vi "DMM Configuration - Update DMM Measurements ComboBox.vi"(8 "error in (no error)":errorcluster, 9 "DMM Temp - Value In":T1={"DMM Temp - Transducer Type"=1, "DMM Temp - Thermocouple Type"=6, "DMM Temp - Fixed Reference Junction"=25.0, "DMM Temp - RTD Type"=enum."Pt3851", "DMM Temp - RTD Resistance"=100.0, "DMM Temp - Thermistor Type"=enum."44006", "DMM Temp - RTD A"=0.0039083, "DMM Temp - RTD B"=-5.775e-07, "DMM Temp - RTD C"=-4.183e-12, "DMM Temp - Thermistor A"=0.0010295, "DMM Temp - Thermistor B"=0.0002391, "DMM Temp - Thermistor C"=1.568e-07} {"DMM Temp - Thermistor C" format="%#_13g"; "DMM Temp - Thermistor B" format="%#_13g"; "DMM Temp - Thermistor A" format="%#_13g"; "DMM Temp - RTD Resistance" format="%.2f"; "DMM Temp - Fixed Reference Junction" format="%.2f"; "DMM Temp - Thermocouple Type" items=["B"=1, "E"=4, "J"=6, "K"=7, "N"=8, "R"=9, "S"=10, "T"=11]; "DMM Temp - Transducer Type" items=["Thermocouple"=1, "Thermistor"=2, "2-Wire RTD"=3, "4-Wire RTD"=4]}, 10 "Measurement In":T7 caption="Function", 11 "Measurement Controls Refs In":T6) -> (0 "error out":errorcluster, 1 "DMM Temp - Value Out":T1={"DMM Temp - Transducer Type"=1, "DMM Temp - Thermocouple Type"=6, "DMM Temp - Fixed Reference Junction"=25.0, "DMM Temp - RTD Type"=enum."Pt3851", "DMM Temp - RTD Resistance"=100.0, "DMM Temp - Thermistor Type"=enum."44006", "DMM Temp - RTD A"=0.0039083, "DMM Temp - RTD B"=-5.775e-07, "DMM Temp - RTD C"=-4.183e-12, "DMM Temp - Thermistor A"=0.0010295, "DMM Temp - Thermistor B"=0.0002391, "DMM Temp - Thermistor C"=1.568e-07} {"DMM Temp - Thermistor C" format="%#_13g"; "DMM Temp - Thermistor B" format="%#_13g"; "DMM Temp - Thermistor A" format="%#_13g"; "DMM Temp - RTD Resistance" format="%.2f"; "DMM Temp - Fixed Reference Junction" format="%.2f"; "DMM Temp - Thermocouple Type" items=["B"=1, "E"=4, "J"=6, "K"=7, "N"=8, "R"=9, "S"=10, "T"=11]; "DMM Temp - Transducer Type" items=["Thermocouple"=1, "Thermistor"=2, "2-Wire RTD"=3, "4-Wire RTD"=4]}, 2 "Temp Meas?":bool, 3 "Measurement Controls Refs Out":T6)   [LabVIEW 2016, in "DMM-SWITCH-ScanList System Explorer.lvlib"]
uses:
  DMM-SWITCH-ScanList System Explorer.lvlib
  <instrlib>/niDMM/nidmm.llb/niDMM Function.ctl
  Configuration Controls/DMM Temp.ctl
  <instrlib>/niDMM/nidmm.llb/niDMM Transducer Type.ctl
  <instrlib>/niDMM/nidmm.llb/niDMM Thermocouple Type.ctl
  <instrlib>/niDMM/nidmm.llb/niDMM RTD Type.ctl
  <instrlib>/niDMM/nidmm.llb/niDMM Thermistor Type.ctl
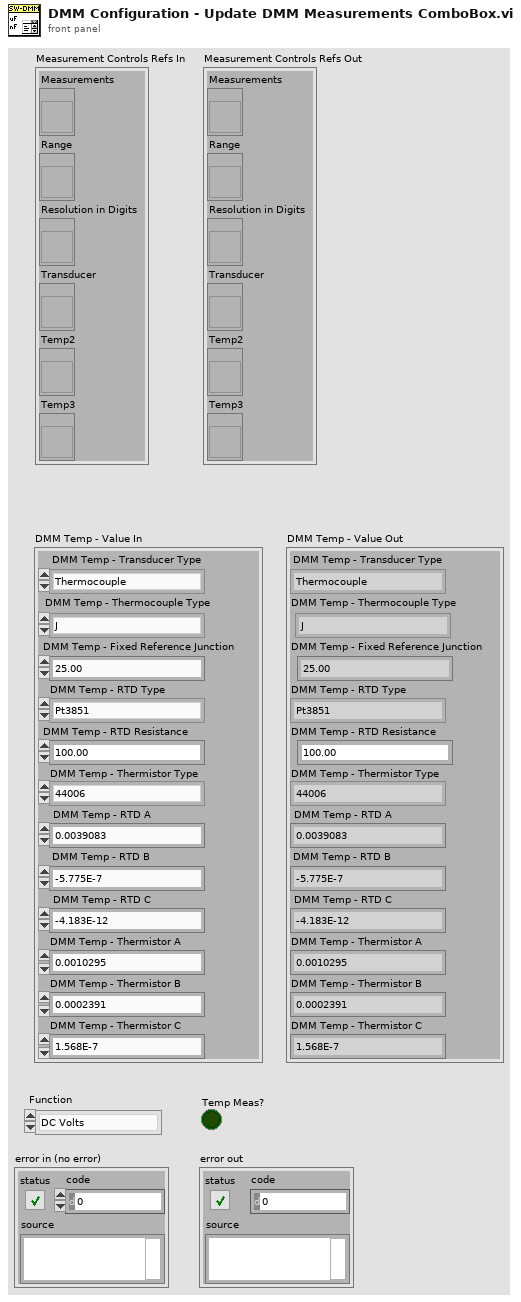
[diagram p1: front panel]
types:
  T1 = typedef "DMM-SWITCH-ScanList System Explorer.lvlib/DMM Temp.ctl" = cluster{"DMM Temp - Transducer Type":T2, "DMM Temp - Thermocouple Type":T3, "DMM Temp - Fixed Reference Junction":dbl, "DMM Temp - RTD Type":T4, "DMM Temp - RTD Resistance":dbl, "DMM Temp - Thermistor Type":T5, "DMM Temp - RTD A":dbl, "DMM Temp - RTD B":dbl, "DMM Temp - RTD C":dbl, "DMM Temp - Thermistor A":dbl, "DMM Temp - Thermistor B":dbl, "DMM Temp - Thermistor C":dbl}
  T2 = typedef "niDMM Transducer Type.ctl" = i32
  T3 = typedef "niDMM Thermocouple Type.ctl" = i32
  T4 = typedef "niDMM RTD Type.ctl" = enum16{"Custom", "Pt3750", "Pt3851", "Pt3911", "Pt3916", "Pt3920", "Pt3928"}
  T5 = typedef "niDMM Thermistor Type.ctl" = enum16{"Custom", "44004", "44006", "44007"}
  T6 = cluster{"Measurements":refnum<vi>, "Range":refnum<vi>, "Resolution in Digits":refnum<vi>, "Transducer":refnum<vi>, "Temp2":refnum<vi>, "Temp3":refnum<vi>}
  T7 = typedef "niDMM Function.ctl" = enum16{"DC Volts", "AC Volts", "DC Current", "AC Current", "2-wire Resistance", "4-wire Resistance", "Diode", "Frequency", "Period", "AC Volts DC Coupled", "Capacitance", "Inductance", "Temperature"}
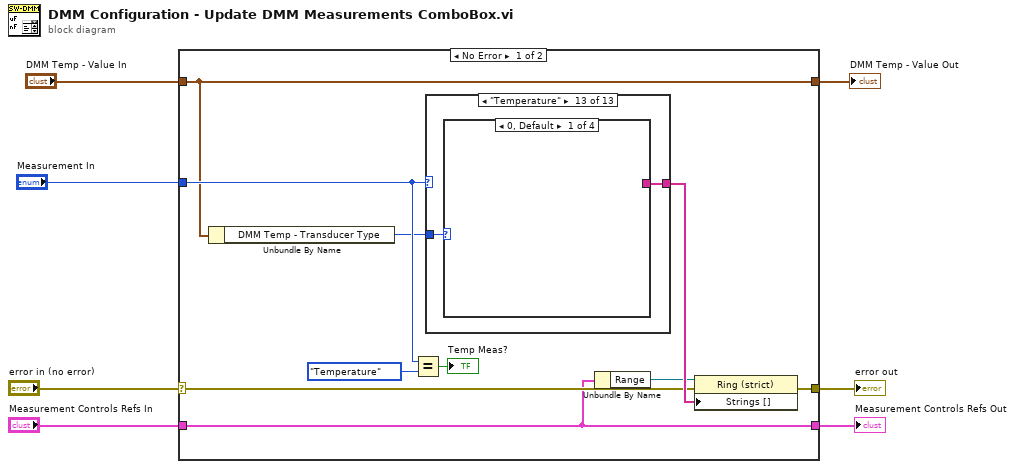
[diagram p0: block diagram]
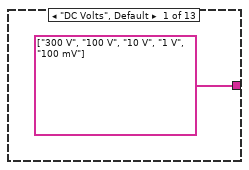
[diagram p2: hidden frame]
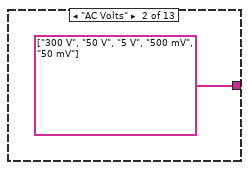
[diagram p3: hidden frame]
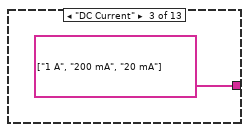
[diagram p4: hidden frame]
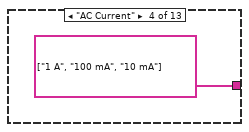
[diagram p5: hidden frame]
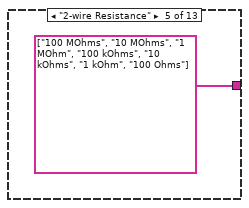
[diagram p6: hidden frame]
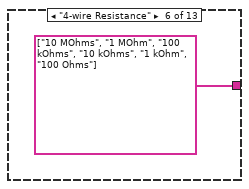
[diagram p7: hidden frame]
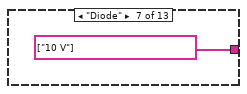
[diagram p8: hidden frame]
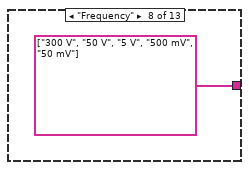
[diagram p9: hidden frame]
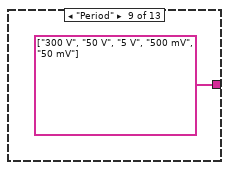
[diagram p10: hidden frame]
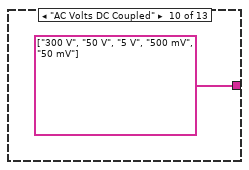
[diagram p11: hidden frame]
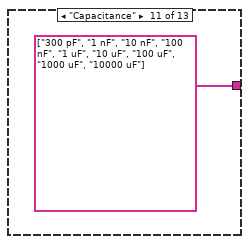
[diagram p12: hidden frame]
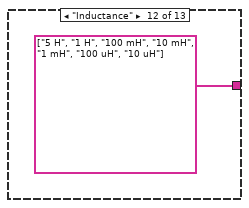
[diagram p13: hidden frame]
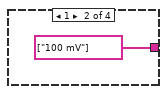
[diagram p14: hidden frame]
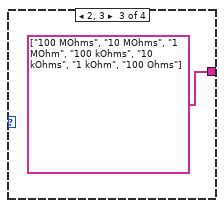
[diagram p15: hidden frame]
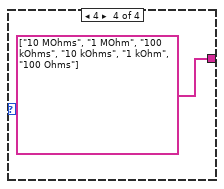
[diagram p16: hidden frame]
diagram:
  n1 = case shown="No Error" "error in (no error)" {
    selector: "error in (no error)" -> [w16 w37]
    tunnel: [w12 w37] -> w7
    tunnel: "Measurement Controls Refs In" -> [w11 w36]
    tunnel: [w11 w36] -> w4
    tunnel: "DMM Temp - Value In" -> [w8 w35]
    tunnel: "Measurement In" -> [w10 _]
    tunnel: [w8 w35] -> w1
    frame No Error {
      n2 = Unbundle By Name(w8) -> ("DMM Temp - Transducer Type"=w9:T2)
      n3 = Equal?(x=w10, y=niDMM_Function."Temperature") -> (x = y?=→"Temp Meas?":bool)
      n4 = case shown="\"Temperature\"" w10 {
        tunnel: [string[] ["300 V", "100 V", "10 V", "1 V", "100 mV"] ("Strings []") string[] ["300 V", "50 V", "5 V", "500 mV", "50 mV"] ("Strings []") string[] ["1 A", "200 mA", "20 mA"] ("Strings []") string[] ["1 A", "100 mA", "10 mA"] ("Strings []") string[] ["100 MOhms", "10 MOhms", "1 MOhm", "100 kOhms", "10 kOhms", "1 kOhm", "100 Ohms"] ("Strings []") string[] ["10 MOhms", "1 MOhm", "100 kOhms", "10 kOhms", "1 kOhm", "100 Ohms"] ("Strings []") string[] ["10 V"] ("Strings []") string[] ["300 V", "50 V", "5 V", "500 mV", "50 mV"] ("Strings []") string[] ["300 V", "50 V", "5 V", "500 mV", "50 mV"] ("Strings []") string[] ["300 V", "50 V", "5 V", "500 mV", "50 mV"] ("Strings []") string[] ["300 pF", "1 nF", "10 nF", "100 nF", "1 uF", "10 uF", "100 uF", "1000 uF", "10000 uF"] ("Strings []") string[] ["5 H", "1 H", "100 mH", "10 mH", "1 mH", "100 uH", "10 uH"] ("Strings []") w31] -> w17
        tunnel: w9 -> [_ _ _ _ _ _ _ _ _ _ _ _ w30]
        frame "DC Volts", Default {
        }
        frame "AC Volts" {
        }
        frame "DC Current" {
        }
        frame "AC Current" {
        }
        frame "2-wire Resistance" {
        }
        frame "4-wire Resistance" {
        }
        frame "Diode" {
        }
        frame "Frequency" {
        }
        frame "Period" {
        }
        frame "AC Volts DC Coupled" {
        }
        frame "Capacitance" {
        }
        frame "Inductance" {
        }
        frame "Temperature" {
          n5 = case shown="0, Default" w30 {
            tunnel: [_ string[] ["100 mV"] string[] ["100 MOhms", "10 MOhms", "1 MOhm", "100 kOhms", "10 kOhms", "1 kOhm", "100 Ohms"] ("Strings []") string[] ["10 MOhms", "1 MOhm", "100 kOhms", "10 kOhms", "1 kOhm", "100 Ohms"] ("Strings []")] -> w31
            frame 0, Default {
            }
            frame 1 {
            }
            frame 2, 3 {
            }
            frame 4 {
            }
          }
        }
      }
      n6 = Unbundle By Name(w11) -> ("Range"=w15:refnum<vi>)
      n7 = property on="Property Node" class="Ring (strict)"(reference=w15, error in=w16, "Strings []"=w17) -> (error out=w12:errorcluster)  [unwired: 1 out]
    }
    frame Error {
    }
  }
  "error out" <- w7
  "Measurement Controls Refs Out" <- w4
  "DMM Temp - Value Out" <- w1
